vi "Get - Time Data OBJ.vi"(0 "reference in":refnum<class "TDMS.lvclass">, 5 "error in (no error)":errorcluster) -> (14 "reference out":refnum<class "TDMS.lvclass">, 16 "Time Data OBJ":refnum<class "GSwFormDSP.lvclass">, 19 "error out":errorcluster)   [LabVIEW 2022 SP3, in "TDMS.lvclass"]
uses:
  TDMS.lvclass
  API/GSwFormDSP_class/GSwFormDSP.lvclass
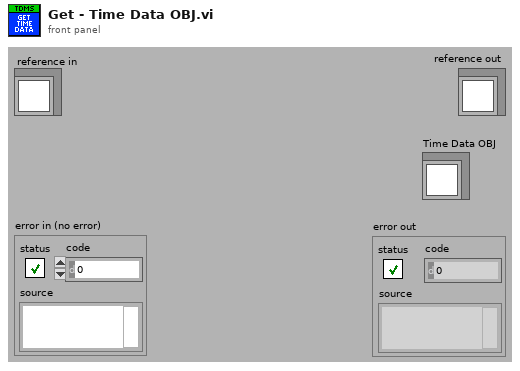
[diagram p1: front panel]
types:
  T1 = typedef "TDMS.lvclass/ObjectAttributes.ctl" = cluster{"Time Data":refnum<class "GSwFormDSP.lvclass">, "New Time Data Obj?":bool}
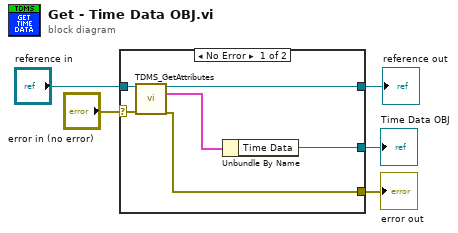
[diagram p0: block diagram]
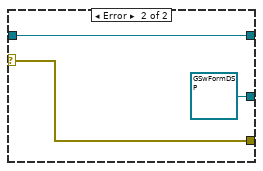
[diagram p2: hidden frame]
diagram:
  n1 = case shown="No Error" "error in (no error)" {
    selector: "error in (no error)" -> [w11 w14]
    tunnel: [w10 w14] -> w4
    tunnel: [w9 w13] -> w2
    tunnel: "reference in" -> [w7 w13]
    tunnel: [w6 refnum<class "GSwFormDSP.lvclass"> refnum ("Time Data")] -> w1
    frame No Error {
      n2 = call "TDMS_GetAttributes.vi"("reference in"=w7, "error in (no error)"=w11) -> ("reference out"=w9:refnum<class "TDMS.lvclass">, "attributes"=w8:T1, "error out"=w10:errorcluster)  [unwired: 14 in, 1 out]
      n3 = Unbundle By Name(w8) -> ("Time Data"=w6:refnum<class "GSwFormDSP.lvclass">)
    }
    frame Error {
    }
  }
  "error out" <- w4
  "reference out" <- w2
  "Time Data OBJ" <- w1
